vi "get_destination.vi"(0 "HGF_Agent.lvclass in":refnum<class "MoAgSy_AgentBase.lvclass">, 5 "error in (no error)":errorcluster) -> (14 "HGF_Agent.lvclass out":refnum<class "MoAgSy_AgentBase.lvclass">, 16 "destination":string, 19 "error out":errorcluster)   [LabVIEW 2009, in "MoAgSy_Base.lvlib" / "MoAgSy_AgentBase.lvclass"]
uses:
  MoAgSy_AgentBase.lvclass
  MoAgSy_AgentBase.lvclass/MoAgSy_AgentBase.ctl
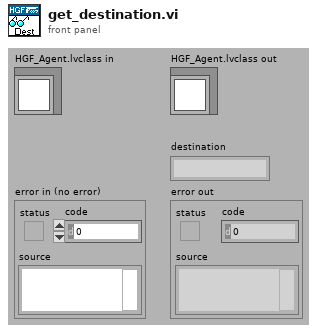
[diagram p1: front panel]
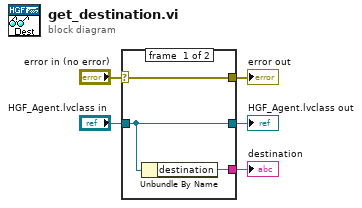
[diagram p0: block diagram]
diagram:
  n1 = case shown="No Error" "error in (no error)" {
    selector: "error in (no error)" -> [w8 w9]
    tunnel: [w8 w9] -> w4
    tunnel: [w7 w10] -> w2
    tunnel: "HGF_Agent.lvclass in" -> [w7 w10]
    tunnel: [w6 _] -> w1
    frame #0 {
      n2 = Unbundle By Name(w7) -> ("destination"=w6:string)
    }
    frame #1 {
    }
  }
  "error out" <- w4
  "HGF_Agent.lvclass out" <- w2
  "destination" <- w1
